vi "Register.vi"(0 "BroadcastRegistry In":T1, 5 "Status":string="status", 7 "Source":string="source", 9 "Api":string="api", 11 "Target":string="target") -> (4 "BroadcastRegistry Out":T1)   [LabVIEW 2017, in "Communicable State Machine.lvlib"]
doc: "### Register.vi\n\n-- <b>Controls</b> --\n- <b>BroadcastRegistry in</b>:\n- <b>status</b>:\n- <b>source</b>:\n- <b>api</b>:\n- <b>target</b>:\n\n-- <b>Indicators</b> --\n- <b>BroadcastRegistry out</b>:"
uses:
  Communicable State Machine.lvlib
  BroadcastRegistry.ctl
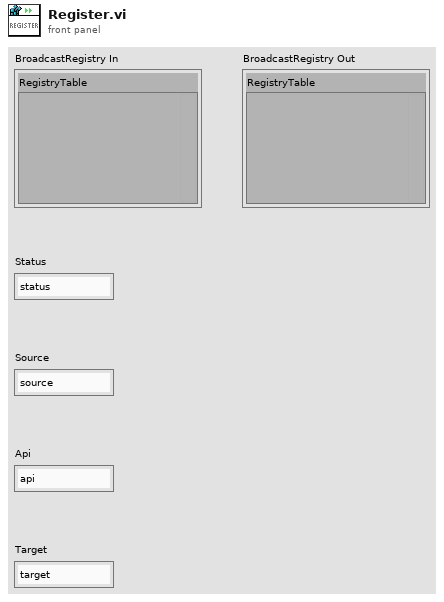
[diagram p1: front panel]
types:
  T1 = typedef "Communicable State Machine.lvlib/BroadcastRegistry.ctl" = cluster{"RegistryTable":variant}
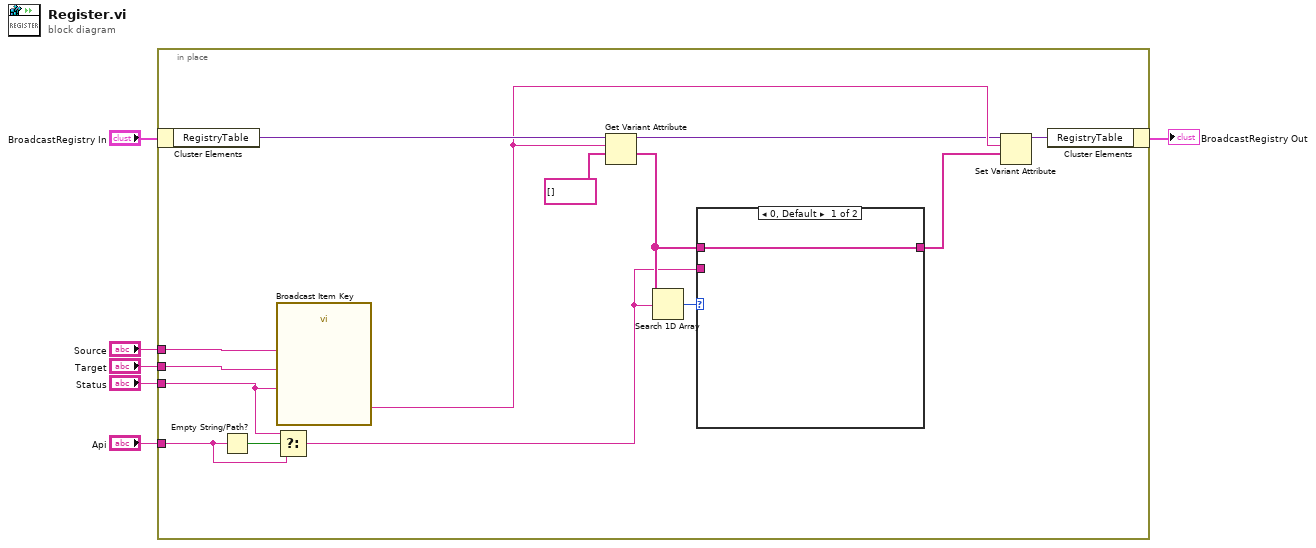
[diagram p0: block diagram]
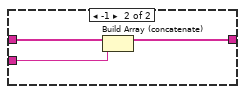
[diagram p2: hidden frame]
diagram:
  n1 = in-place {
    in-place-border: "Status" -> [w19]
    in-place-border: "Target" -> [w18]
    in-place-border: "Source" -> [w17]
    in-place-border: "Api" -> [w16]
    n2 = in-place-cluster #1("BroadcastRegistry In") -> ("RegistryTable"=w15:variant)
    n3 = Empty String/Path?(string/path=w16) -> (empty?=w20:bool)
    n4 = call "Broadcast Item Key.vi"("Status"=w19, "Target"=w18, "Source"=w17) -> ("Key"=w14:string)  [unwired: 2 in]
    n5 = Select(t=w19, s=w20, f=w16) -> (s? t:f=w7:string)
    n6 = Get Variant Attribute(Variant=w15, name=w14, default value (empty Variant)=string[] [] ("output cluster")) -> (duplicate Variant=w11:variant, value=w9:string[])  [unwired: 1 in, 2 out]
    n7 = Search 1D Array(1D array=w9, element=w7) -> (index of element=w12:i32)  [unwired: 1 in]
    n8 = case shown="0, Default" w12 {
      tunnel: w9 -> [w21 w24]
      tunnel: [w21 w23] -> w8
      tunnel: w7 -> [_ w22]
      frame 0, Default {
      }
      frame -1 {
        n9 = Build Array (concatenate)(w24, w22) -> (w23:string[])
      }
    }
    n10 = Set Variant Attribute(Variant=w11, name=w14, value=w8) -> (Variant out=w13:variant)  [unwired: 1 in, 2 out]
    n11 = in-place-cluster #1("RegistryTable"=w13) -> (→"BroadcastRegistry Out":T1)
  }
